vi "LimitChange.vi"(9 "Previous Output":dbl=nan, 10 "Ramp (1/s)":dbl, 11 "Set Point":dbl) -> (3 "Output":dbl)   [LabVIEW 2015]
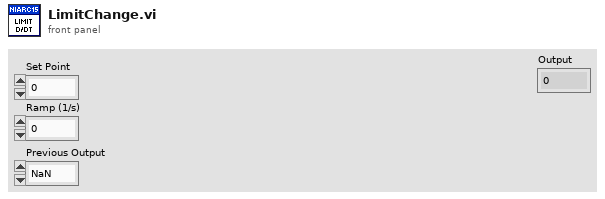
[diagram p1: front panel]
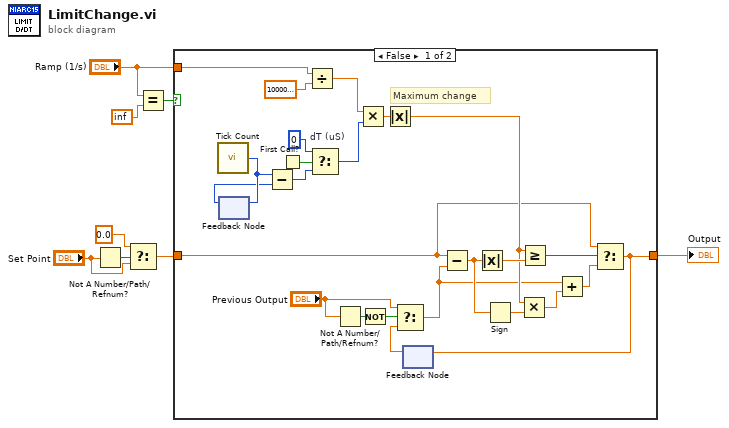
[diagram p0: block diagram]
diagram:
  n1 = Not A Number/Path/Refnum?(number/path/refnum="Set Point") -> (NaN/Path/Refnum?=w7:bool)
  n2 = Select(t=0.0, s=w7, f="Set Point") -> (s? t:f=w6:dbl)
  n3 = Equal?(x="Ramp (1/s)", y=inf) -> (x = y?=w3:bool)
  n4 = case shown="False" w3 {
    tunnel: "Ramp (1/s)" -> [w29 _]
    tunnel: [w10 w33] -> w8
    tunnel: w6 -> [w9 w33]
    frame False {
      # "Maximum change"
      n5 = call "Tick Count"() -> ("Tick Count(uSec)"=w32:u32)
      n6 = feedback #1() -> (w31:u32)  [unwired: 1 in]
      n7 = feedback-in #1(w32) -> ()
      n8 = Subtract(x=w32, y=w31) -> (x-y=w26:u32)
      n9 = First Call?() -> (First Call?: T/F=w30:bool)
      n10 = Divide(x=w29, y=1000000.0) -> (x/y=w23:dbl)
      n11 = Select "dT (uS)"(t=u32 0, s=w30, f=w26) -> (s? t:f=w24:u32)
      n12 = Not A Number/Path/Refnum?(number/path/refnum="Previous Output") -> (NaN/Path/Refnum?=w15:bool)
      n13 = Multiply(x=w23, y=w24) -> (x*y=w27:dbl)
      n14 = Not(x=w15) -> (.not. x?=w14:bool)
      n15 = Absolute Value(x=w27) -> (abs(x)=w17:dbl)
      n16 = feedback #2() -> (w11:dbl)  [unwired: 1 in]
      n17 = Select(t="Previous Output", s=w14, f=w11) -> (s? t:f=w12:dbl)
      n18 = Subtract(x=w9, y=w12) -> (x-y=w22:dbl)
      n19 = Absolute Value(x=w22) -> (abs(x)=w20:dbl)
      n20 = Sign(1:w22) -> (0:w18:dbl)
      n21 = Multiply(x=w17, y=w18) -> (x*y=w16:dbl)
      n22 = Greater Or Equal?(x=w17, y=w20) -> (x >= y?=w21:bool)
      n23 = Add(x=w12, y=w16) -> (x+y=w19:dbl)
      n24 = Select(t=w9, s=w21, f=w19) -> (s? t:f=w10:dbl)
      n25 = feedback-in #2(w10) -> ()
    }
    frame True {
    }
  }
  "Output" <- w8
